vi "New Interface.vi"(7 "id (0)":i32, 8 "error in (no error)":errorcluster, 9 "fifo options":T3, 10 "fifo descriptors":T1={"command fifo"={"fifo depth"=10, "element size"=0}, "response fifo"={"fifo depth"=10, "element size"=0}, "error fifo"={"fifo depth"=10, "element size"=0}} {"error fifo"."element size" format="%d bytes"; "response fifo"."element size" format="%d bytes"; "command fifo"."element size" format="%d bytes"}, 11 "Interface type":refnum<class "Interface.lvclass">) -> (0 "error out":errorcluster, 3 "Interface":refnum<class "Interface.lvclass">)   [LabVIEW 2019, in "DSF Core.lvlib" / "Interface.lvclass"]
uses:
  Interface.lvclass
  Typedefs/DSF FIFO Options.ctl
  FIFO Descriptors.ctl
  FIFO Descriptor.ctl
  Interface.lvclass/Interface.ctl
  Framework/Framework.lvclass
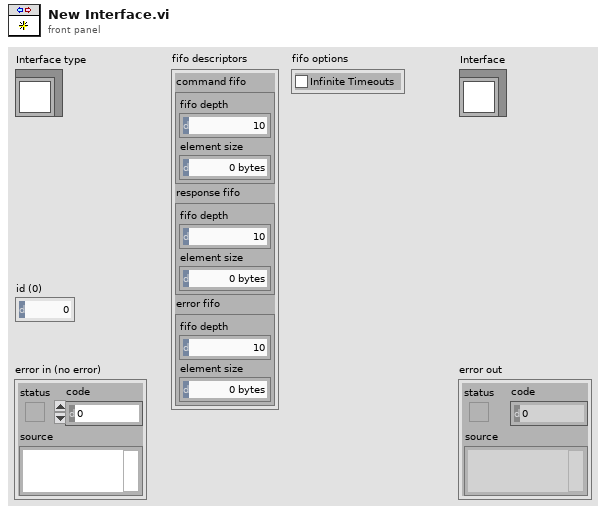
[diagram p1: front panel]
types:
  T1 = typedef "DSF Core.lvlib/Interface.lvclass/FIFO Descriptors.ctl" = cluster{"command fifo":T2, "response fifo":T2, "error fifo":T2}
  T2 = typedef "DSF Core.lvlib/Interface.lvclass/FIFO Descriptor.ctl" = cluster{"fifo depth":u32, "element size":u32}
  T3 = typedef "DSF Core.lvlib/Framework.lvclass/DSF FIFO Options.ctl" = cluster{"Infinite Timeouts":bool}
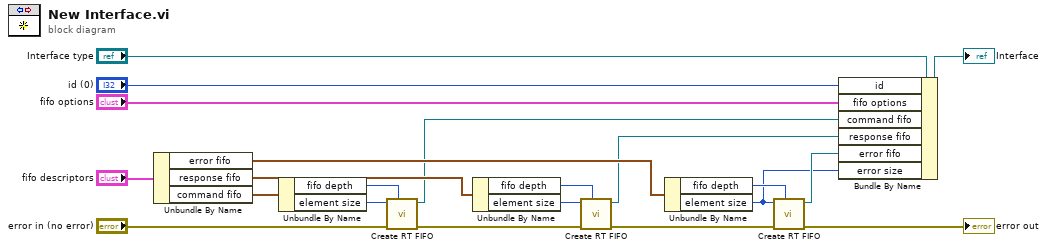
[diagram p0: block diagram]
diagram:
  n1 = Unbundle By Name("fifo descriptors") -> ("error fifo"=w4:T2, "response fifo"=w5:T2, "command fifo"=w11:T2)
  n2 = Unbundle By Name(w11) -> ("fifo depth"=w9:u32, "element size"=w10:u32)
  n3 = call "Create RT FIFO.vi"("fifo depth (10)"=w9, "error in (no error)"="error in (no error)", "element size"=w10) -> ("error out"=w16:errorcluster, "rt fifo"=w3:refnum<k33>)  [unwired: 7 in]
  n4 = Unbundle By Name(w5) -> ("fifo depth"=w7:u32, "element size"=w8:u32)
  n5 = call "Create RT FIFO.vi"("fifo depth (10)"=w7, "error in (no error)"=w16, "element size"=w8) -> ("error out"=w15:errorcluster, "rt fifo"=w2:refnum<k33>)  [unwired: 7 in]
  n6 = Unbundle By Name(w4) -> ("fifo depth"=w6:u32, "element size"=w1:u32)
  n7 = call "Create RT FIFO.vi"("fifo depth (10)"=w6, "error in (no error)"=w15, "element size"=w1) -> ("error out"=→"error out":errorcluster, "rt fifo"=w13:refnum<k33>)  [unwired: 7 in]
  n8 = Bundle By Name(cluster="Interface type", "id"="id (0)", "fifo options"="fifo options", "command fifo"=w3, "response fifo"=w2, "error fifo"=w13, "error size"=w1) -> (→"Interface":refnum<class "Interface.lvclass">)
